vi "Rec Fetch Next Recordset (CR).vi"(4 "error in (no error)":errorcluster, 7 "command-recordset reference":T1) -> (0 "error out":errorcluster, 3 "command-recordset reference out":T1)   [LabVIEW 2020, in "NI_Database_API.lvlib"]
doc: "Retrieves the next recordset in a multi-recordset query identified by <B>recordset reference</B>. When the current recordset is no longer available, the <B>recordset reference</B> is redirected to the new recordset. Wire data to the reference input to determine the polymorphic instance to use or manually select the instance."
uses:
  <vilib>/addons/database/NI_Database_API.lvlib
  <vilib>/addons/database/Command-Recordset.llb/Cmd-Rec Object Reference.ctl
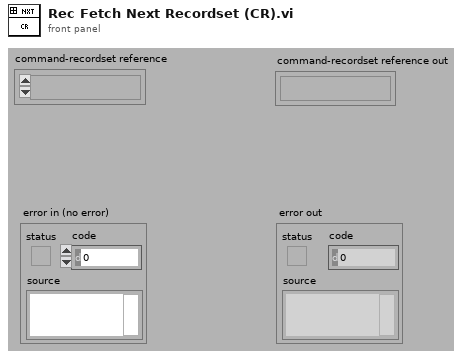
[diagram p1: front panel]
types:
  T1 = typedef "NI_Database_API.lvlib/Cmd-Rec Object Reference.ctl" = refnum<k1>
  T2 = typedef "NI_Database_API.lvlib/Cmd-Rec Data Members.ctl" = cluster{"recordset reference":T3, "command reference":T4}
  T3 = typedef "NI_Database_API.lvlib/Rec ObjectReference.ctl" = refnum<k1>
  T4 = typedef "NI_Database_API.lvlib/Cmd ObjectReference.ctl" = refnum<k1>
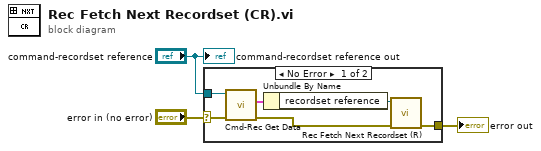
[diagram p0: block diagram]
diagram:
  n1 = case shown="No Error" "error in (no error)" {
    selector: "error in (no error)" -> [w4 w10]
    tunnel: [w9 w10] -> w3
    tunnel: "command-recordset reference" -> [w5 _]
    frame No Error {
      n2 = call <vilib>:"Cmd-Rec Get Data.vi"("error in (no error)"=w4, "command-recordset reference"=w5) -> ("error out"=w6:errorcluster, "data"=w7:T2)  [unwired: 2 in, 2 out]
      n3 = Unbundle By Name(w7) -> ("recordset reference"=w8:T3)
      n4 = call <vilib>:"Rec Fetch Next Recordset (R).vi"("error in (no error)"=w6, "recordset reference"=w8) -> ("error out"=w9:errorcluster)  [unwired: 4 in, 1 out]
    }
    frame Error {
    }
  }
  "error out" <- w3
  "command-recordset reference out" <- "command-recordset reference"
